vi "Close.vi"(8 "error in (no error)":errorcluster caption="错误输入（无错误）", 11 "5720A 输入":refnum<class "5720A.lvclass">) -> (0 "error out":errorcluster caption="错误输出", 3 "5720A 输出":refnum<class "5720A.lvclass">)   [LabVIEW 2020, in "5720A.lvlib" / "5720A.lvclass"]
uses:
  5720A.lvclass
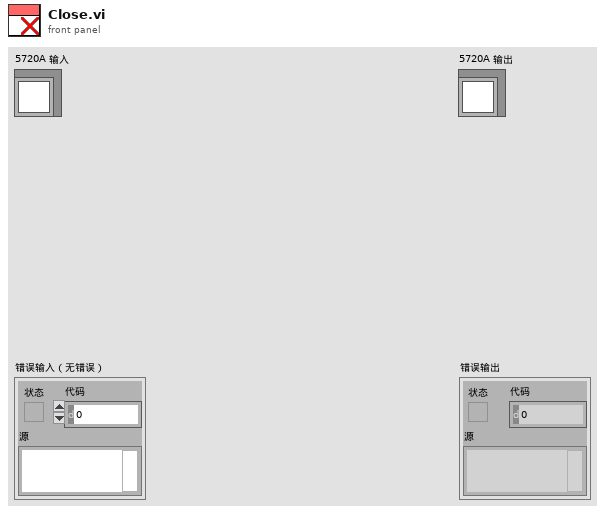
[diagram p1: front panel]
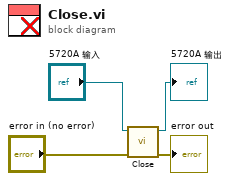
[diagram p0: block diagram]
diagram:
  n1 = call-parent "Close.vi"("error in (no error)"="error in (no error)", "多功能校准源接口 输入"="5720A 输入") -> ("error out"=→"error out":errorcluster, "多功能校准源接口 输出"=→"5720A 输出":refnum<class "5720A.lvclass">)  [unwired: 8 in]
